vi "Create or Access Log Path.vi"(8 "error in":errorcluster, 11 "Module Data In":refnum<class "Rename.lvclass">) -> (0 "error out":errorcluster, 1 "Log Path":path, 2 "Log Refnum Out":refnum<file>, 3 "Module Data Out":refnum<class "Rename.lvclass">)   [LabVIEW 2015, in "Generic Module Library.lvlib" / "Template G_Module.lvlib"]
uses:
  Template G_Module.lvlib
  <vilib>/Utility/sysdir.llb/System Directory Type.ctl
  Module Class/Rename.lvclass
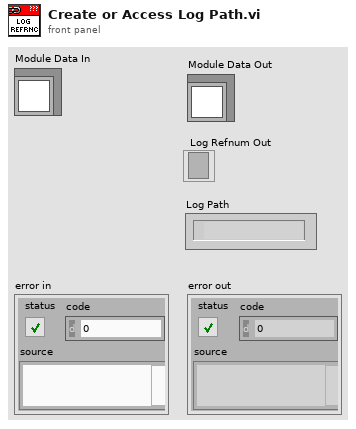
[diagram p1: front panel]
types:
  T1 = enum16{"open", "replace", "create", "open or create", "replace or create", "replace or create with confirmation"}
  T2 = typedef "System Directory Type.ctl" = i32
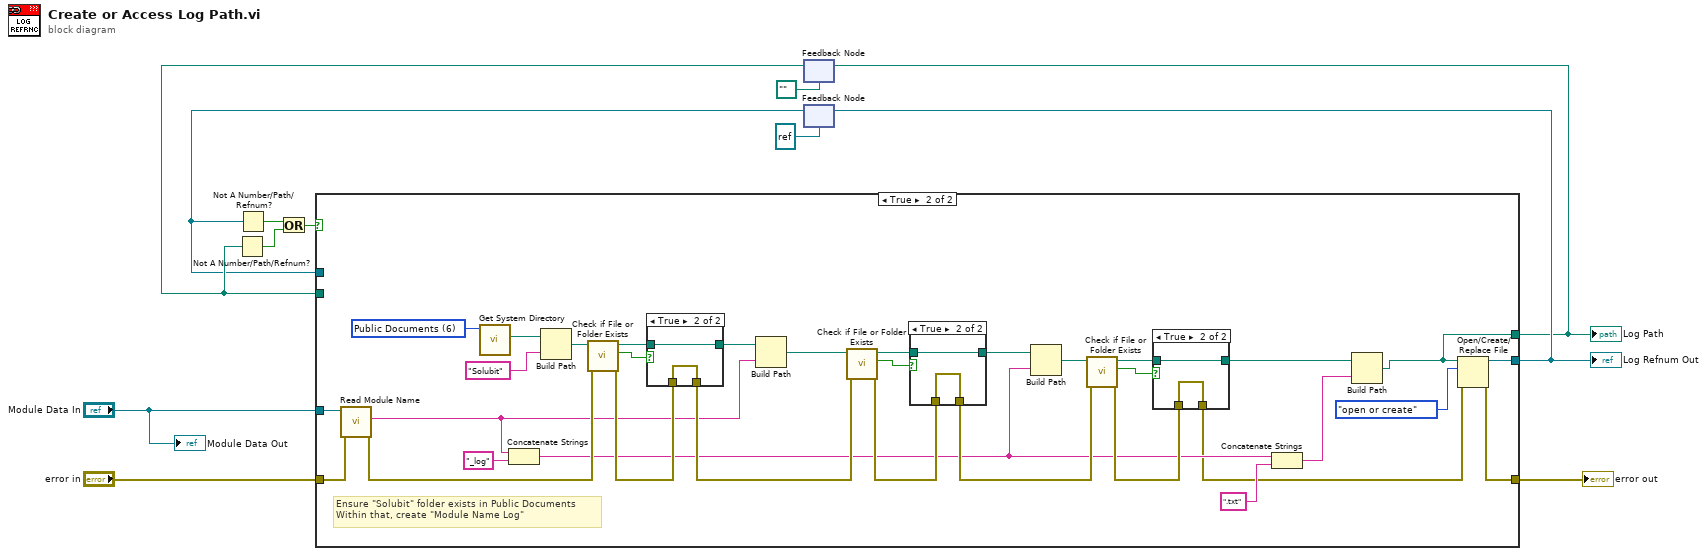
[diagram p0: block diagram]
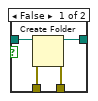
[diagram p3: hidden frame]
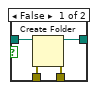
[diagram p4: hidden frame]
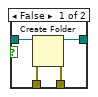
[diagram p5: hidden frame]
diagram:
  n1 = feedback #1(path "" ("appended path")) -> (w5:path)
  n2 = Not A Number/Path/Refnum?(number/path/refnum=w5) -> (NaN/Path/Refnum?=w1:bool)
  n3 = feedback #2(refnum<file> refnum ("refnum out")) -> (w4:refnum<file>)
  n4 = Not A Number/Path/Refnum?(number/path/refnum=w4) -> (NaN/Path/Refnum?=w2:bool)
  n5 = Or(x=w2, y=w1) -> (x .or. y?=w3:bool)
  n6 = case shown="True" w3 {
    tunnel: "Module Data In" -> [_ w41]
    tunnel: "error in" -> [w15 w40]
    tunnel: [w15 w17] -> w12
    tunnel: [w14 w24] -> w9
    tunnel: w4 -> [w14 _]
    tunnel: [w13 w16] -> w8
    tunnel: w5 -> [w13 _]
    frame False {
    }
    frame True {
      w48 = T2 6 items=["User Home"=0, "User Desktop"=1, "User Documents"=2, "User Application Data"=3, "User Preferences"=4, "User Temporary"=5, "Public Documents"=6, "Public Application Data"=7, "Public Preferences"=8, "Public Cache"=13, "System Core Libraries"=9, "System Installed Libraries"=10, "Application Files"=11, "Boot Volume Root"=12] ("system directory type")
      # "Ensure \"Solubit\" folder exists in Public Documents\nWithin that, create \"Module Name Log\""
      n7 = call-dynamic "Read Module Name.vi"("error in (no error)"=w40, "Rename in"=w41) -> ("error out"=w26:errorcluster, "Module Name"=w25:string)  [unwired: 7 in, 1 out]
      n8 = call <vilib>:"Get System Directory.vi"("system directory type"=w48) -> ("system directory"=w47:path)  [unwired: 10 in]
      n9 = Concatenate Strings(w25, "_log" ("string")) -> (w22:string)
      n10 = Build Path(base path=w47, name or relative path="Solubit") -> (appended path=w45:path)
      n11 = call <vilib>:"Check if File or Folder Exists.vi"("error in (no error)"=w26, "path"=w45) -> ("error out"=w42:errorcluster, "file or folder exists?"=w43:bool, "dup path"=w44:path)  [unwired: 7 in]
      n12 = case shown="True" w43 {
        tunnel: w44 -> [w58 w60]
        tunnel: w42 -> [w57 w59]
        tunnel: [w55 w59] -> w36
        tunnel: [w56 w60] -> w38
        frame False {
          n13 = Create Folder(path (use dialog)=w58, error in=w57) -> (created path=w56:path, error out=w55:errorcluster)  [unwired: 1 in, 1 out]
        }
        frame True {
        }
      }
      n14 = Build Path(base path=w38, name or relative path=w25) -> (appended path=w37:path)
      n15 = call <vilib>:"Check if File or Folder Exists.vi"("error in (no error)"=w36, "path"=w37) -> ("error out"=w33:errorcluster, "file or folder exists?"=w34:bool, "dup path"=w35:path)  [unwired: 7 in]
      n16 = case shown="True" w34 {
        tunnel: w35 -> [w52 w54]
        tunnel: w33 -> [w51 w53]
        tunnel: [w49 w53] -> w32
        tunnel: [w50 w54] -> w31
        frame False {
          n17 = Create Folder(path (use dialog)=w52, error in=w51) -> (created path=w50:path, error out=w49:errorcluster)  [unwired: 1 in, 1 out]
        }
        frame True {
        }
      }
      n18 = Build Path(base path=w31, name or relative path=w22) -> (appended path=w27:path)
      n19 = call <vilib>:"Check if File or Folder Exists.vi"("error in (no error)"=w32, "path"=w27) -> ("error out"=w28:errorcluster, "file or folder exists?"=w29:bool, "dup path"=w30:path)  [unwired: 7 in]
      n20 = case shown="True" w29 {
        tunnel: w30 -> [w64 w66]
        tunnel: w28 -> [w63 w65]
        tunnel: [w62 w65] -> w18
        tunnel: [w61 w66] -> w23
        frame False {
          n21 = Create Folder(path (use dialog)=w64, error in=w63) -> (created path=w61:path, error out=w62:errorcluster)  [unwired: 1 in, 1 out]
        }
        frame True {
        }
      }
      n22 = Concatenate Strings(w22, ".txt" ("string")) -> (w20:string)
      n23 = Build Path(base path=w23, name or relative path=w20) -> (appended path=w16:path)
      n24 = Open/Create/Replace File(file path (use dialog)=w16, error in=w18, operation (0:open)=T1."open or create") -> (refnum out=w24:refnum<file>, error out=w17:errorcluster)  [unwired: 3 in, 1 out]
    }
  }
  "error out" <- w12
  "Log Refnum Out" <- w9
  "Log Path" <- w8
  n25 = feedback-in #1(w8) -> ()
  n26 = feedback-in #2(w9) -> ()
  "Module Data Out" <- "Module Data In"
